vi "Change Network Settings.vi"(6 "Execution State in":T1, 7 "Deploy in":enum16{"Deploy", "Troubleshoot"}(ring), 8 "error in (no error)":errorcluster, 9 "Network Settings in":T2, 10 "Targets in":T4 {"Filtered Targets"."IP Mode" items=["Static"=1, "DHCP/Link-Local"=2, "Link-Local Only"=4, "DHCP Only"=8]}, 11 "Ctl Refs in":T7) -> (0 "error out":errorcluster, 1 "Network Settings out":T2, 2 "Targets out":T4 {"Filtered Targets"."IP Mode" items=["Static"=1, "DHCP/Link-Local"=2, "Link-Local Only"=4, "DHCP Only"=8]}, 3 "Ctl Refs out":T7, 4 "Buttons out":T3, 5 "Execution State out":T1)   [LabVIEW 2013]
uses:
  Controls/Refs.ctl
  Controls/Button Refs.ctl
  Controls/Tab Ctl Refs.ctl
  types/TabStateType.ctl
  Controls/Indicator Refs.ctl
  Controls/Slider Refs.ctl
  Controls/Control Refs.ctl
  Controls/Targets.ctl
  Controls/Detected.ctl
  types/MAX Sys Cfg Target Information.ctl
  types/ButtonStateType.ctl
  Controls/Network Settings.ctl
  types/ExecutionStateType.ctl
  <vilib>/nisyscfg/Initialize (String).vi
  <vilib>/nisyscfg/Close (System).vi
  <vilib>/nisyscfg/nisyscfg.lvlib
  <resource>/objmgr/nisysapi.rc
panel:
  in  "stop_loop":bool
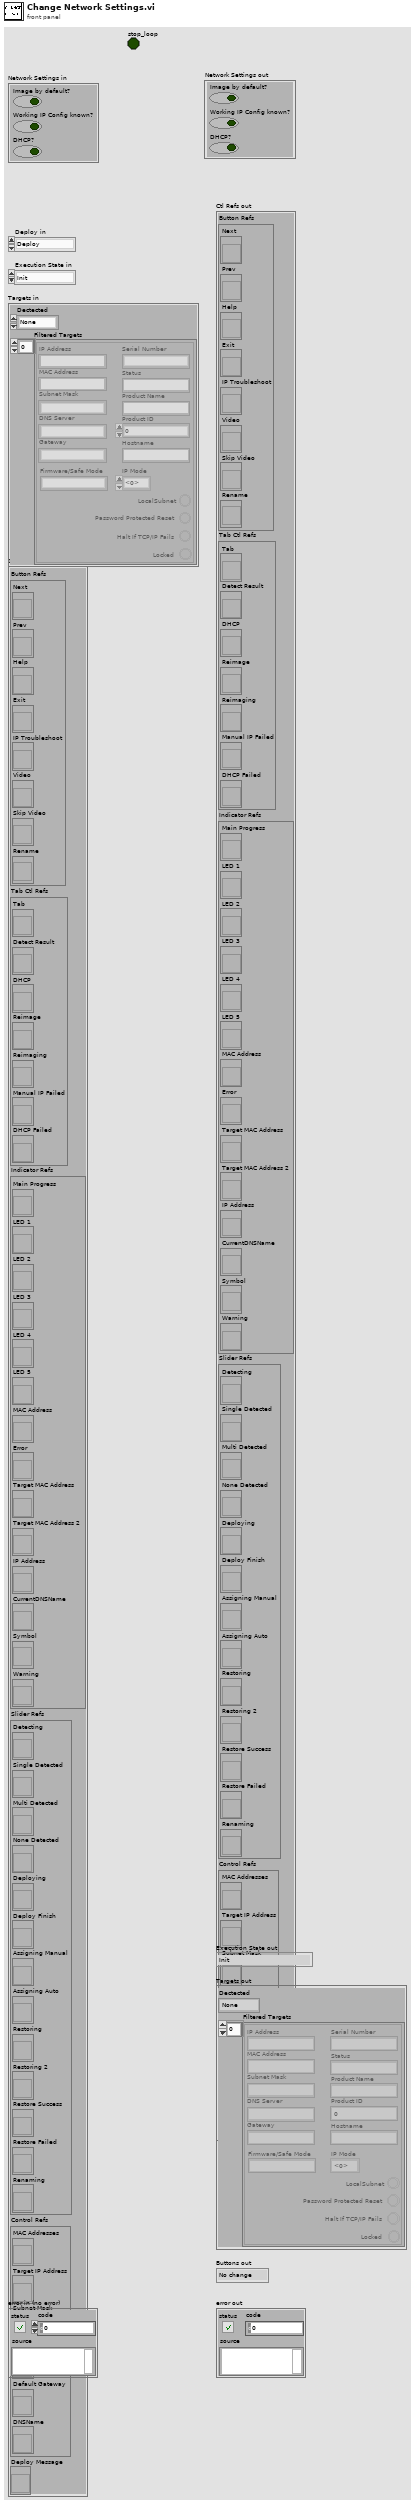
[diagram p1: front panel]
types:
  T1 = typedef "ExecutionStateType.ctl" = enum16{"Init", "Welcome", "Idle", "Detect", "Run Detection", "Detect Fail", "Detect One", "Detect Mult", "Deploy", "DHCP", "Static IP", "Run Deployment", "Connect Verify", "Exit", "Video Wait", "Success", "Troubleshoot", "Troubleshoot 2", "RenameDNS"}
  T2 = typedef "Network Settings.ctl" = cluster{"Image by default?":bool, "Working IP Config known?":bool, "DHCP?":bool}
  T3 = typedef "ButtonStateType.ctl" = enum16{"No change", "No Next", "No Prev", "All Disabled", "All Enabled", "Exit Only"}
  T4 = typedef "Targets.ctl" = cluster{"Dectected":T5, "Filtered Targets":T6[]}
  T5 = typedef "Detected.ctl" = enum16{"None", "Failed", "Single", "Multi"}
  T6 = typedef "MAX Sys Cfg Target Information.ctl" = cluster{"MAC Address":string, "IP Address":string, "Status":string, "Product Name":string, "Hostname":string, "Firmware/Safe Mode":string, "Subnet Mask":string, "Gateway":string, "DNS Server":string, "Serial Number":string, "Product ID":u32, "Locked ":bool, "LocalSubnet":bool, "Halt If TCP/IP Fails":bool, "Password Protected Reset":bool, "IP Mode":i32}
  T7 = typedef "Refs.ctl" = cluster{"Button Refs":T8, "Tab Ctl Refs":T9, "Indicator Refs":T10, "Slider Refs":T11, "Control Refs":T12, "Deploy Message":refnum<vi>}
  T8 = typedef "Button Refs.ctl" = cluster{"Next":refnum<vi>, "Prev":refnum<vi>, "Help":refnum<vi>, "Exit":refnum<vi>, "IP Troubleshoot":refnum<vi>, "Video":refnum<vi>, "Skip Video":refnum<vi>, "Rename":refnum<vi>}
  T9 = typedef "Tab Ctl Refs.ctl" = cluster{"Tab":refnum<vi>, "Detect Result":refnum<vi>, "DHCP":refnum<vi>, "Reimage":refnum<vi>, "Reimaging":refnum<vi>, "Manual IP Failed":refnum<vi>, "DHCP Failed":refnum<vi>}
  T10 = typedef "Indicator Refs.ctl" = cluster{"Main Progress":refnum<vi>, "LED 1":refnum<vi>, "LED 2":refnum<vi>, "LED 3":refnum<vi>, "LED 4":refnum<vi>, "LED 5":refnum<vi>, "MAC Address":refnum<vi>, "Error":refnum<vi>, "Target MAC Address":refnum<vi>, "Target MAC Address 2":refnum<vi>, "IP Address":refnum<vi>, "CurrentDNSName":refnum<vi>, "Symbol":refnum<vi>, "Warning":refnum<vi>}
  T11 = typedef "Slider Refs.ctl" = cluster{"Detecting":refnum<vi>, "Single Detected":refnum<vi>, "Multi Detected":refnum<vi>, "None Detected":refnum<vi>, "Deploying":refnum<vi>, "Deploy Finish":refnum<vi>, "Assigning Manual":refnum<vi>, "Assigning Auto":refnum<vi>, "Restoring":refnum<vi>, "Restoring 2":refnum<vi>, "Restore Success":refnum<vi>, "Restore Failed":refnum<vi>, "Renaming":refnum<vi>}
  T12 = typedef "Control Refs.ctl" = cluster{"MAC Addresses":refnum<vi>, "Target IP Address":refnum<vi>, "Subnet Mask":refnum<vi>, "DNS IP":refnum<vi>, "Default Gateway":refnum<vi>, "DNSName":refnum<vi>}
  T13 = cluster{"Value":string, "Value":string, "Value":string, "Value":string}
  T14 = cluster{"Image by default?":bool, bool, "Use DHCP (True)?":bool}
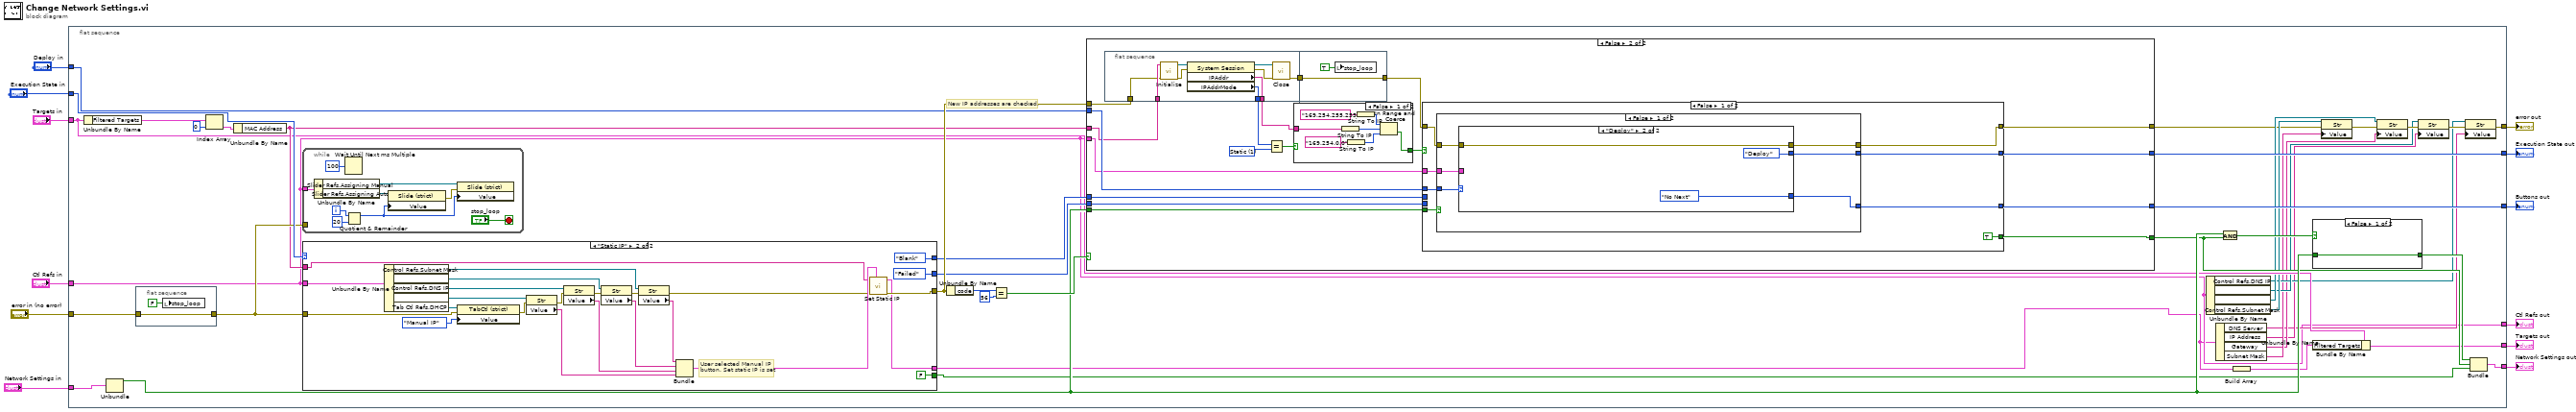
[diagram p0: block diagram]
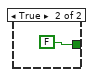
[diagram p2: hidden frame]
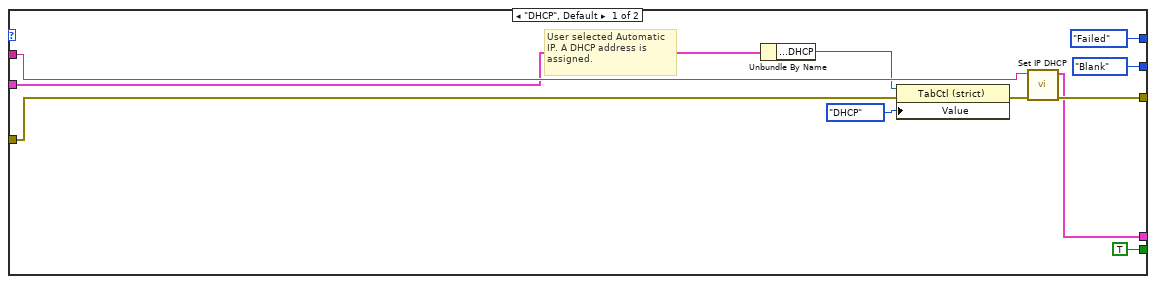
[diagram p3: hidden frame]
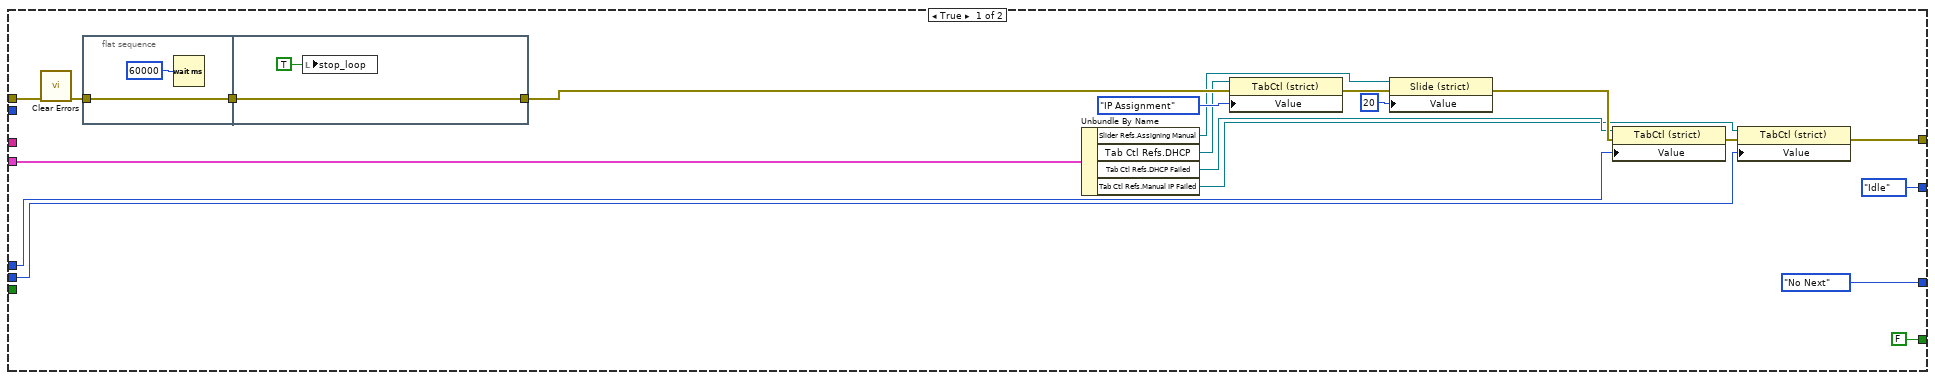
[diagram p4: hidden frame]
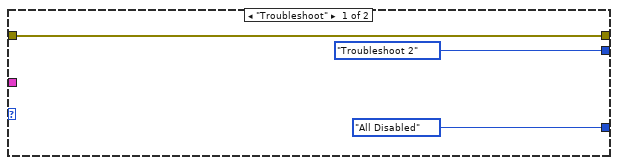
[diagram p6: hidden frame]
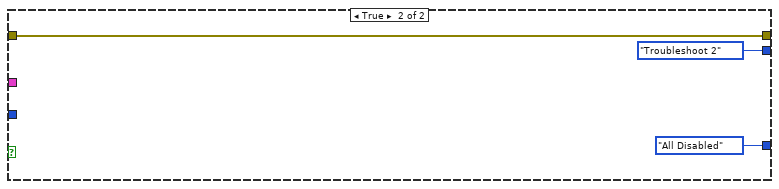
[diagram p7: hidden frame]
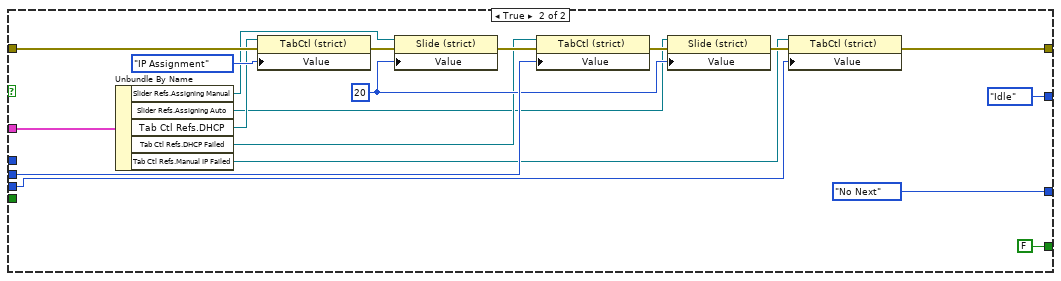
[diagram p8: hidden frame]
diagram:
  n1 = flat-sequence {
    tunnel: "error in (no error)" -> [w52]
    tunnel: "Deploy in" -> [w46]
    tunnel: [w45] -> w3
    tunnel: [w44] -> w4
    tunnel: "Execution State in" -> [w43]
    tunnel: "Network Settings in" -> [w42]
    tunnel: [w37] -> w7
    tunnel: "Targets in" -> [w31]
    tunnel: [w29] -> w9
    tunnel: [w19] -> w10
    tunnel: "Ctl Refs in" -> [w15]
    tunnel: [w15] -> w12
    frame #0 {
      # "New IP addresses are checked."
      n2 = Unbundle By Name(w31) -> ("Filtered Targets"=w32:T6[])
      n3 = Unbundle(w42) -> ("Image by default?"=w35:bool)  [unwired: 2 out]
      n4 = flat-sequence {
        tunnel: w52 -> [w203]
        tunnel: [w203] -> w39
        frame #0 {
          n5 = local write "stop_loop"(FALSE ("stop_loop")) -> ()
        }
      }
      n6 = Index Array(array=w32, index=0) -> (element=w53:T6)
      n7 = Unbundle By Name(w53) -> ("MAC Address"=w33:string)
      n8 = while {
        tunnel: w39 -> [_]
        tunnel: w15 -> [w198]
        i -> [w199]
        stop <- "stop_loop" stop-if-true
        n9 = Unbundle By Name(w198) -> ("Slider Refs.Assigning Manual"=w195:refnum<vi>, "Slider Refs.Assigning Auto"=w197:refnum<vi>)
        n10 = Wait Until Next ms Multiple(millisecond multiple=u32 100 ("milliseconds to wait")) -> ()  [unwired: 1 out]
        n11 = Quotient & Remainder(x=w199, y=20) -> (x-y*floor(x/y)=w194:i32)  [unwired: 1 out]
        n12 = property class="Slide (strict)"(reference=w197, "Value"=w194) -> (error out=w196:errorcluster)  [unwired: 1 in, 1 out]
        n13 = property class="Slide (strict)"(reference=w195, error in=w196, "Value"=w194) -> ()  [unwired: 2 out]
      }
      n14 = case shown="\"Static IP\"" w43 {
        tunnel: [w59 w83] -> w47
        tunnel: w39 -> [w64 w90]
        tunnel: w33 -> [w61 w84]
        tunnel: [w56 w67] -> w13
        tunnel: [enum32{"Failed", "Blank"}."Failed" ("DHCP Failed Tab") enum32{"Failed", "Blank"}."Blank" ("DHCP Failed Tab")] -> w41
        tunnel: [enum32{"Failed", "Blank"}."Blank" ("Manual IP Failed Tab") enum32{"Failed", "Blank"}."Failed" ("Manual IP Failed Tab")] -> w40
        tunnel: [TRUE ("Use DHCP (True)?") FALSE ("Use DHCP (True)?")] -> w14
        tunnel: w15 -> [w57 w82]
        frame "DHCP", Default {
          # "User selected Automatic\nIP. A DHCP address is\nassigned."
          n15 = Unbundle By Name(w57) -> ("Tab Ctl Refs.DHCP"=w58:refnum<vi>)
          n16 = property on="Property Node" class="TabCtl (strict)"(reference=w58, error in=w64, "Value"=enum32{"IP Assignment", "DHCP", "Manual IP"}."DHCP" ("DHCP Tabs")) -> (error out=w60:errorcluster)  [unwired: 1 out]
          n17 = call "Set IP DHCP.vi"("error in"=w60, "MAC Address"=w61) -> ("error out"=w59:errorcluster, "Network Module Information"=w56:T6)  [unwired: 8 in]
        }
        frame "Static IP" {
          # "User selected Manual IP\nbutton. Set static IP is set"
          n18 = Unbundle By Name(w82) -> ("Control Refs.Subnet Mask"=w69:refnum<vi>, "Control Refs.Default Gateway"=w74:refnum<vi>, "Control Refs.DNS IP"=w76:refnum<vi>, "Control Refs.Target IP Address"=w79:refnum<vi>, "Tab Ctl Refs.DHCP"=w81:refnum<vi>)
          n19 = property on="Property Node" class="TabCtl (strict)"(reference=w81, error in=w90, "Value"=enum32{"IP Assignment", "DHCP", "Manual IP"}."Manual IP" ("DHCP Tabs")) -> (error out=w80:errorcluster)  [unwired: 1 out]
          n20 = property class="Str"(reference=w79, error in=w80) -> (error out=w78:errorcluster, "Value"=w77:string)  [unwired: 1 out]
          n21 = property class="Str"(reference=w76, error in=w78) -> (error out=w73:errorcluster, "Value"=w75:string)  [unwired: 1 out]
          n22 = property class="Str"(reference=w74, error in=w73) -> (error out=w70:errorcluster, "Value"=w72:string)  [unwired: 1 out]
          n23 = property class="Str"(reference=w69, error in=w70) -> (error out=w71:errorcluster, "Value"=w68:string)  [unwired: 1 out]
          n24 = Bundle("Value"=w68, "Value"=w72, "Value"=w75, "Value"=w77) -> (w85:T13)  [unwired: 1 out]
          n25 = call "Set Static IP.vi"("MAC Address"=w84, "error in (no error)"=w71, "Target Info In"=w85) -> ("Network Module Information"=w67:T6, "error out"=w83:errorcluster)  [unwired: 6 in]
        }
      }
      n26 = Unbundle By Name(w47) -> ("code"=w50:i32)
      n27 = Equal?(x=w50, y=56) -> (x = y?=w48:bool)
      n28 = case shown="False" w48 {
        tunnel: w47 -> [w110 w127]
        tunnel: [w102 w132] -> w20
        tunnel: w46 -> [_ w131]
        tunnel: [ExecutionStateType."Idle" ("Enum") w130] -> w45
        tunnel: w33 -> [_ w128]
        tunnel: [FALSE w125] -> w34
        tunnel: w35 -> [_ w124]
        tunnel: w41 -> [w99 w123]
        tunnel: w40 -> [w98 w122]
        tunnel: [ButtonStateType."No Next" ("Enum") w121] -> w37
        tunnel: w15 -> [w95 w119]
        frame True {
          n29 = call <vilib>:"Clear Errors.vi"("error in (no error)"=w110) -> ("error out"=w106:errorcluster)  [unwired: 6 out]
          n30 = flat-sequence {
            tunnel: w106 -> [w112]
            tunnel: [w112] -> w97
            tunnel: [w114] -> w105
            tunnel: w97 -> [w114]
            frame #0 {
              n31 = Wait (ms)(milliseconds to wait=u32 60000) -> ()  [unwired: 1 out]
            }
            frame #1 {
              n32 = local write "stop_loop"(TRUE ("stop_loop")) -> ()
            }
          }
          n33 = Unbundle By Name(w95) -> ("Slider Refs.Assigning Manual"=w91:refnum<vi>, "Tab Ctl Refs.DHCP"=w94:refnum<vi>, "Tab Ctl Refs.DHCP Failed"=w93:refnum<vi>, "Tab Ctl Refs.Manual IP Failed"=w92:refnum<vi>)
          n34 = property on="Property Node" class="TabCtl (strict)"(reference=w94, error in=w105, "Value"=enum32{"IP Assignment", "DHCP", "Manual IP"}."IP Assignment" ("DHCP Tabs")) -> (error out=w109:errorcluster)  [unwired: 1 out]
          n35 = property on="Property Node" class="Slide (strict)"(reference=w91, error in=w109, "Value"=i8 20 ("Slide 7")) -> (error out=w104:errorcluster)  [unwired: 1 out]
          n36 = property on="Property Node" class="TabCtl (strict)"(reference=w93, error in=w104, "Value"=w99) -> (error out=w103:errorcluster)  [unwired: 1 out]
          n37 = property on="Property Node" class="TabCtl (strict)"(reference=w92, error in=w103, "Value"=w98) -> (error out=w102:errorcluster)  [unwired: 1 out]
        }
        frame False {
          w115 = 1 items=["Static"=1, "DHCP/Link-Local"=2, "Link-Local Only"=4, "DHCP Only"=8] ("Primary NIC:IP Address Request Mode")
          n38 = flat-sequence {
            tunnel: w128 -> [w188]
            tunnel: [w186] -> w129
            tunnel: w127 -> [w187]
            tunnel: [w183] -> w120
            tunnel: [w182] -> w117
            tunnel: [w192] -> w126
            tunnel: w129 -> [w192]
            frame #0 {
              n39 = call-poly <vilib>:"Initialize.vi"("error in (no error)"=w187, "target (localhost)"=w188) -> ("error out"=w189:errorcluster, "session out"=w185:refnum<k21>)  [unwired: 7 in, 1 out]
              n40 = property class="System Session"(reference=w185, error in=w189) -> (reference out=w184:refnum<k21>, error out=w190:errorcluster, "IPAddr"=w183:string, "IPAddrMode"=w182:i32)
              n41 = call-poly <vilib>:"Close.vi"("error in (no error)"=w190, "session in"=w184) -> ("error out"=w186:errorcluster)  [unwired: 9 in]
            }
            frame #1 {
              n42 = local write "stop_loop"(TRUE ("stop_loop")) -> ()
            }
          }
          n43 = Equal?(x=w117, y=w115) -> (x = y?=w116:bool)
          n44 = case shown="False" w116 {
            tunnel: w120 -> [w134 _]
            tunnel: [w133 _] -> w118
            frame False {
              n45 = String To IP(1:w134) -> (0:w135:u32)
              n46 = String To IP(1:"169.254.0.0" ("name")) -> (0:w136:u32)
              n47 = String To IP(1:"169.254.255.255" ("name")) -> (0:w137:u32)
              n48 = In Range and Coerce(upper limit=w137, x=w135, lower limit=w136) -> (In Range?=w133:bool)  [unwired: 1 out]
            }
            frame True {
            }
          }
          n49 = case shown="False" w118 {
            tunnel: [w147 w171] -> w132
            tunnel: w131 -> [w141 _]
            tunnel: [w146 ExecutionStateType."Idle" ("Enum")] -> w130
            tunnel: w126 -> [w145 w179]
            tunnel: [TRUE FALSE] -> w125
            tunnel: w124 -> [w143 _]
            tunnel: w123 -> [_ w175]
            tunnel: w122 -> [_ w174]
            tunnel: [w142 ButtonStateType."No Next" ("Enum")] -> w121
            tunnel: w119 -> [w140 w168]
            frame False {
              n50 = case shown="False" w143 {
                tunnel: [w153 w160] -> w147
                tunnel: w141 -> [w152 _]
                tunnel: [w151 ExecutionStateType."Troubleshoot 2" ("Enum")] -> w146
                tunnel: w145 -> [w150 w160]
                tunnel: [w149 ButtonStateType."All Disabled" ("Enum")] -> w142
                tunnel: w140 -> [w148 _]
                frame False {
                  n51 = case shown="\"Deploy\"" w152 {
                    tunnel: [w155 w157] -> w153
                    tunnel: [ExecutionStateType."Troubleshoot 2" ("Enum") ExecutionStateType."Deploy" ("Enum")] -> w151
                    tunnel: w150 -> [w155 w157]
                    tunnel: [ButtonStateType."All Disabled" ("Enum") ButtonStateType."No Next" ("Enum")] -> w149
                    tunnel: w148 -> [_ _]
                    frame "Troubleshoot" {
                    }
                    frame "Deploy" {
                    }
                  }
                }
                frame True {
                }
              }
            }
            frame True {
              w170 = i8 20 ("Slide 7")
              n52 = Unbundle By Name(w168) -> ("Slider Refs.Assigning Manual"=w164:refnum<vi>, "Slider Refs.Assigning Auto"=w163:refnum<vi>, "Tab Ctl Refs.DHCP"=w167:refnum<vi>, "Tab Ctl Refs.DHCP Failed"=w166:refnum<vi>, "Tab Ctl Refs.Manual IP Failed"=w165:refnum<vi>)
              n53 = property on="Property Node" class="TabCtl (strict)"(reference=w167, error in=w179, "Value"=enum32{"IP Assignment", "DHCP", "Manual IP"}."IP Assignment" ("DHCP Tabs")) -> (error out=w178:errorcluster)  [unwired: 1 out]
              n54 = property on="Property Node" class="Slide (strict)"(reference=w164, error in=w178, "Value"=w170) -> (error out=w177:errorcluster)  [unwired: 1 out]
              n55 = property on="Property Node" class="TabCtl (strict)"(reference=w166, error in=w177, "Value"=w175) -> (error out=w173:errorcluster)  [unwired: 1 out]
              n56 = property on="Property Node" class="Slide (strict)"(reference=w163, error in=w173, "Value"=w170) -> (error out=w172:errorcluster)  [unwired: 1 out]
              n57 = property on="Property Node" class="TabCtl (strict)"(reference=w165, error in=w172, "Value"=w174) -> (error out=w171:errorcluster)  [unwired: 1 out]
            }
          }
        }
      }
      n58 = Unbundle By Name(w15) -> ("Control Refs.DNS IP"=w22:refnum<vi>, "Control Refs.Target IP Address"=w23:refnum<vi>, "Control Refs.Default Gateway"=w24:refnum<vi>, "Control Refs.Subnet Mask"=w25:refnum<vi>)
      n59 = Unbundle By Name(w13) -> ("DNS Server"=w16:string, "IP Address"=w17:string, "Gateway"=w18:string, "Subnet Mask"=w21:string)
      n60 = And(x=w35, y=w34) -> (x .and. y?=w36:bool)
      n61 = Build Array(w13) -> (w30:T6[])
      n62 = case shown="False" w36 {
        tunnel: [w54 FALSE] -> w38
        tunnel: w35 -> [w54 _]
        frame False {
        }
        frame True {
        }
      }
      n63 = Bundle By Name(cluster=w31, "Filtered Targets"=w30) -> (w29:T4)
      n64 = property class="Str"(reference=w25, error in=w20, "Value"=w21) -> (error out=w26:errorcluster)  [unwired: 1 out]
      n65 = property class="Str"(reference=w24, error in=w26, "Value"=w18) -> (error out=w27:errorcluster)  [unwired: 1 out]
      n66 = property class="Str"(reference=w23, error in=w27, "Value"=w17) -> (error out=w28:errorcluster)  [unwired: 1 out]
      n67 = property class="Str"(reference=w22, error in=w28, "Value"=w16) -> (error out=w19:errorcluster)  [unwired: 1 out]
      n68 = Bundle("Image by default?"=w38, w34, "Use DHCP (True)?"=w14) -> (w44:T14)  [unwired: 1 out]
    }
  }
  "Ctl Refs out" <- w12
  "error out" <- w10
  "Targets out" <- w9
  "Buttons out" <- w7
  "Network Settings out" <- w4
  "Execution State out" <- w3
